vi "FM_pll.vi"() -> ()   [LabVIEW 2013]
uses:
  <vilib>/addons/Modulation/Analog/MT Passband PLL.vi
  <vilib>/sound2/lvsound2.llb/Sound File Info (path).vi
  <vilib>/sound2/lvsound2.llb/Sound File Read Open.vi
  <vilib>/sound2/lvsound2.llb/Sound File Read (DBL).vi
  <vilib>/Waveform/WDTOps.llb/WDT Get Waveform Subset DBL.vi
  <vilib>/express/express analysis/Spectral/Block/exnSpectralBlock spectral measurements RMS poly.vi
  <vilib>/express/express analysis/Spectral/Block/exnSpectralBlock spectral measurements RMS DDT.vi
  <vilib>/express/express analysis/Spectral/XNode/ExpressSpectralMeasurementsBlockNode.xnode
  <vilib>/addons/Modulation/niAMT.lvlib
  <vilib>/Analysis/NI_AALPro.lvlib
panel:
  in  "Modulated Signal Source":enum32{"Single Tone", "From File"}(tab)
  in  "ST Frequency":dbl=2000.0 caption="Frequency"
  in  "ST Amplitude":dbl=1.0 caption="Amplitude"
  in  "Resample Rate":dbl=1000000.0 format="%#_6f"
  in  "Duration":dbl=44100.0
  in  "WAV Path":path=path "E:/07/0409/mozart.wav" caption="Path"
  in  "Normalized Peak Amplitude":dbl=1.0 caption="Peak Amplitude"
  out "Estimated Freq.":dbl=100000.0 caption="Frequency"
  in  "WAV Sample Rate":dbl=44100.0 caption="dt"
  in  "LPF Cut-Off":dbl=20000.0 caption="Lower Cut-Off"
  in  "SNR (dB)":dbl(slide)=30.0 caption="Standard deviation" scale=-20.0..50.0
  out "Recovered Signal":dynamicdata(graph)
  out "Baseband":dynamicdata(graph)
  out "FM FFT":dynamicdata(graph)
  out "FM Wave":dynamicdata(graph)
  in  "Carrier Amp.":dbl=1.0 caption="Amplitude"
  in  "stop":bool
  in  "k_f":dbl(slide)=20000.0 scale=0.0..50000.0
  in  "Carrier Freq.":dbl=100000.0 caption="Frequency"
  # "Frequency Modulation"
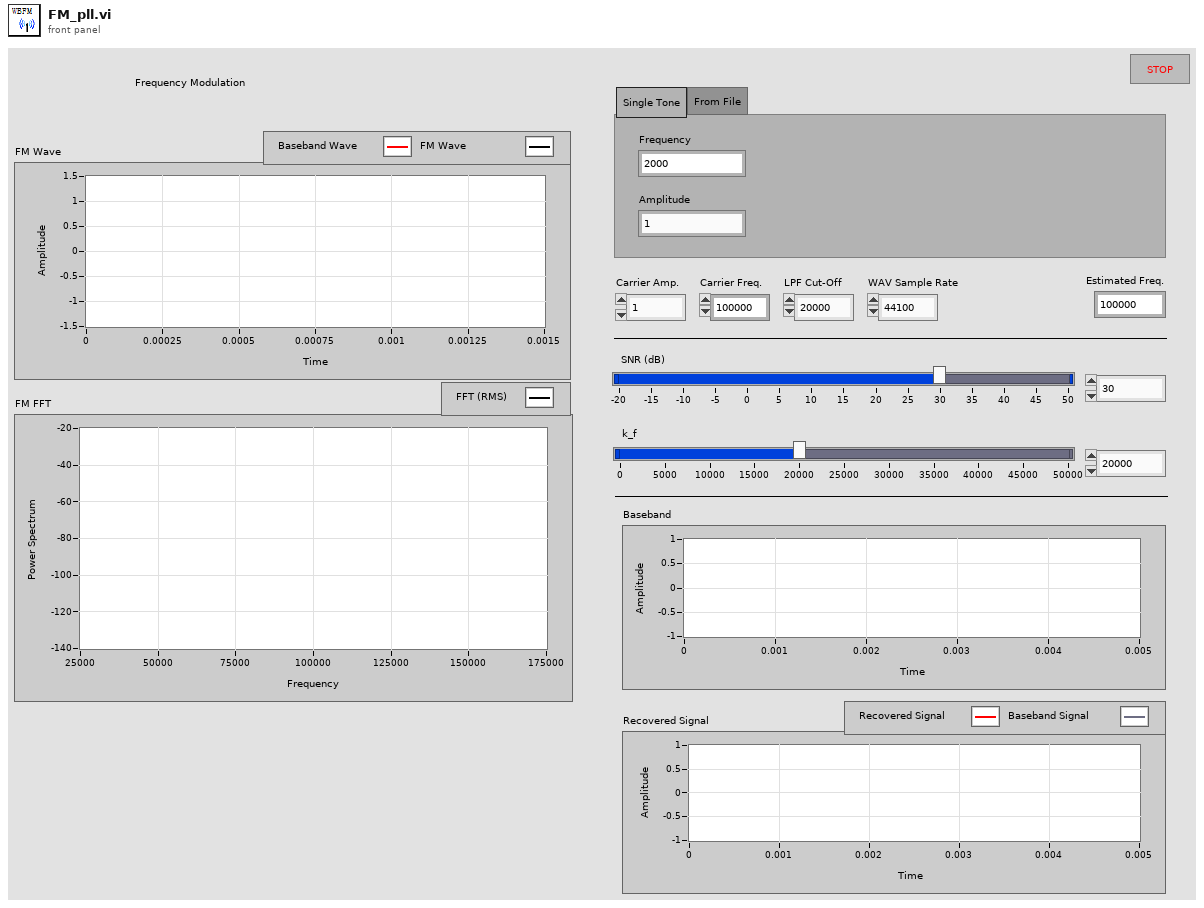
[diagram p1: front panel]
types:
  T1 = cluster{"averaging mode":u16, "weighting mode":u16, "number of averages":u32}
  T2 = cluster{"dB On (F)":bool, "unwrap phase (F)":bool, "convert to degree (F)":bool}
  T3 = typedef "Sound File Refnum.ctl" = refnum<file>
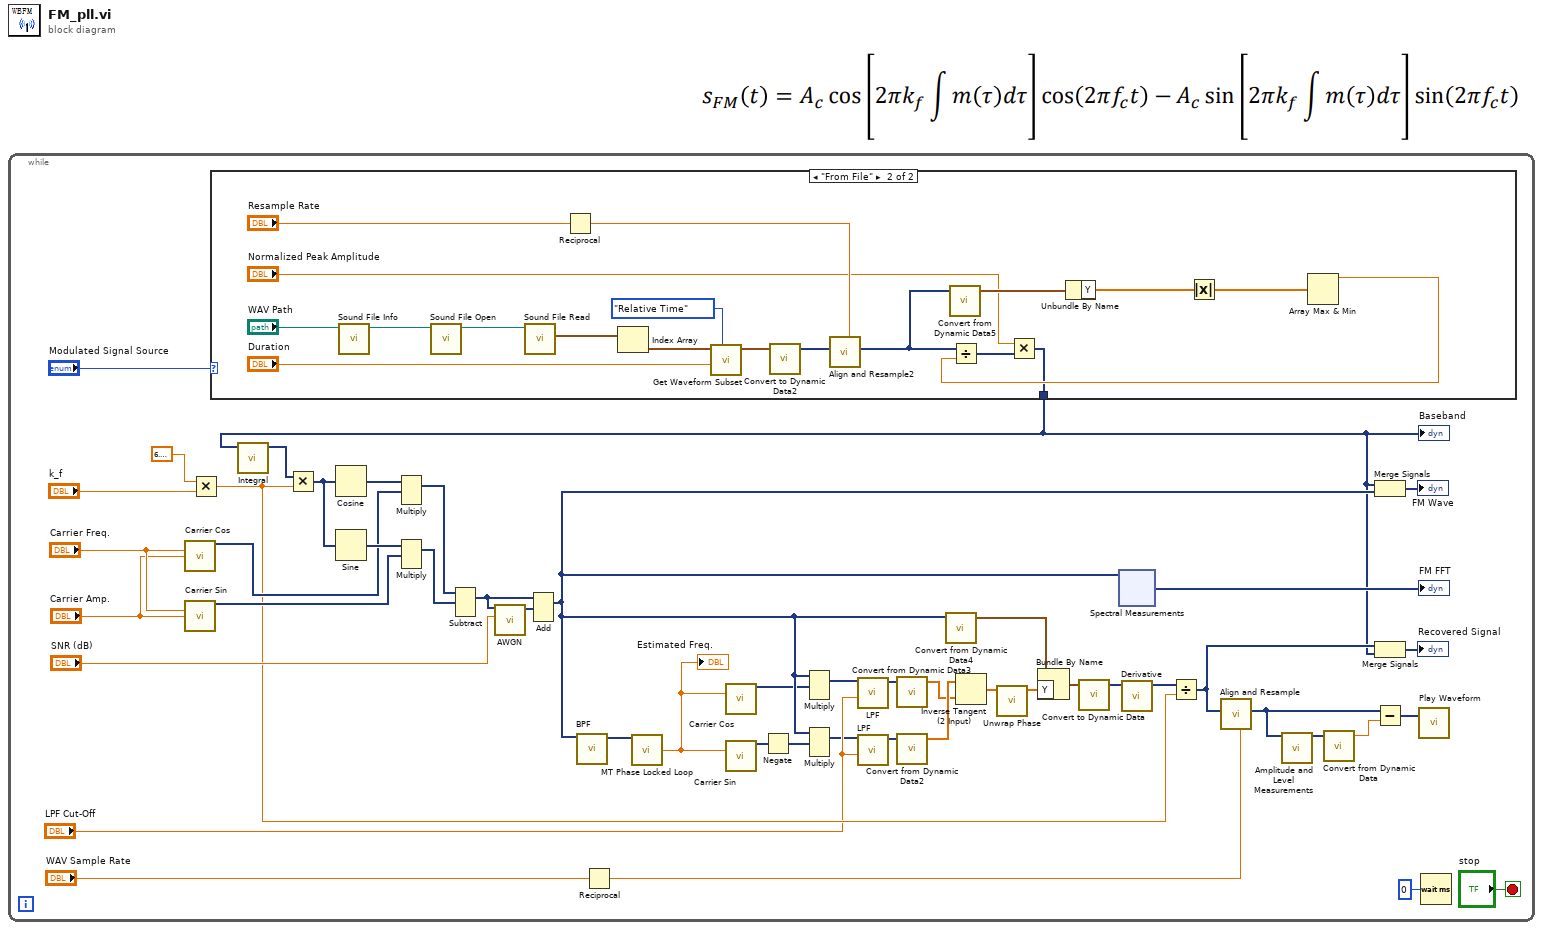
[diagram p0: block diagram]
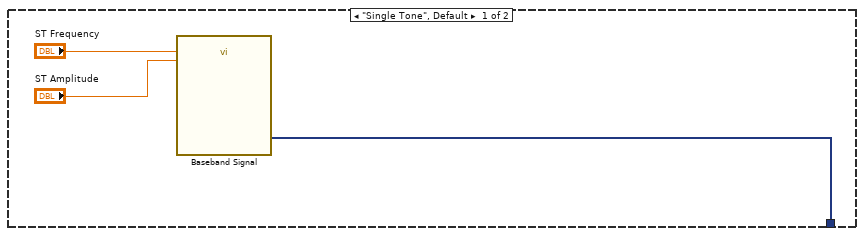
[diagram p2: hidden frame]
diagram:
  n1 = while {
    stop <- "stop" stop-if-true
    n2 = call "Carrier Cos"("Frequency"="Carrier Freq.", "Amplitude"="Carrier Amp.") -> ("Sine"=w28:dynamicdata)  [unwired: 12 in, 1 out]
    n3 = call "Carrier Sin"("Frequency"="Carrier Freq.", "Amplitude"="Carrier Amp.") -> ("Sine"=w27:dynamicdata)  [unwired: 12 in, 1 out]
    n4 = Multiply(x=6.283185307179586, y="k_f") -> (x*y=w23:dbl)
    n5 = case shown="\"From File\"" "Modulated Signal Source" {
      tunnel: [w50 w54] -> w1
      frame "Single Tone", Default {
        n6 = call "Baseband Signal"("Frequency"="ST Frequency", "Amplitude"="ST Amplitude") -> ("Sine"=w50:dynamicdata)  [unwired: 12 in, 1 out]
      }
      frame "From File" {
        n7 = call-poly <vilib>:"Sound File Info.vi"("path"="WAV Path") -> ("path out"=w69:path)  [unwired: 7 in, 3 out]
        n8 = call-poly <vilib>:"Sound File Open.vi"("path"=w69) -> ("sound file refnum"=w71:T3)  [unwired: 9 in, 1 out]
        n9 = call-poly <vilib>:"Sound File Read.vi"("sound file refnum"=w71) -> ("data"=w66:waveform(dbl)[])  [unwired: 6 in, 4 out]
        n10 = Reciprocal(x="Resample Rate") -> (1/x=w62:dbl)
        n11 = Index Array(array=w66) -> (element=w67:waveform(dbl))  [unwired: 1 in]
        n12 = call-poly <vilib>:"Get Waveform Subset.vi"("start/duration format"=enum16{"Relative Time"}."Relative Time", "duration"="Duration", "waveform in"=w67) -> ("waveform out"=w61:waveform(dbl))  [unwired: 3 in, 3 out]
        n13 = call "Convert to Dynamic Data2"("Waveform"=w61) -> ("Dynamic Data Type"=w56:dynamicdata)  [unwired: 3 in]
        n14 = call "Align and Resample2"("dt"=w62, "Signals"=w56) -> ("Resampled Signals"=w57:dynamicdata)  [unwired: 7 in, 2 out]
        n15 = call "Convert from Dynamic Data5"("Dynamic Data Type"=w57) -> ("Waveform"=w64:waveform(dbl))  [unwired: 3 in]
        n16 = Unbundle By Name(w64) -> ("Y"=w58:dbl[])
        n17 = Absolute Value(x=w58) -> (abs(x)=w60:dbl[])
        n18 = Array Max & Min(array=w60) -> (max value=w59:dbl)  [unwired: 3 out]
        n19 = Divide(x=w57, y=w59) -> (x/y=w55:dynamicdata)
        n20 = Multiply(x="Normalized Peak Amplitude", y=w55) -> (x*y=w54:dynamicdata)
      }
    }
    "Baseband" <- w1
    n21 = call "Integral"("Signals"=w1) -> ("Result"=w2:dynamicdata)  [unwired: 5 in, 1 out]
    n22 = Multiply(x=w2, y=w23) -> (x*y=w32:dynamicdata)
    n23 = Cosine(x=w32) -> (cos(x)=w34:dynamicdata)
    n24 = Sine(x=w32) -> (sin(x)=w33:dynamicdata)
    n25 = Multiply(1:w28, 2:w34) -> (0:w30:dynamicdata)  [unwired: 1 in, 1 out]
    n26 = Multiply(1:w27, 2:w33) -> (0:w29:dynamicdata)  [unwired: 1 in, 1 out]
    n27 = Subtract(1:w29, 2:w30) -> (0:w31:dynamicdata)  [unwired: 1 in, 1 out]
    n28 = call "AWGN.vi"("SNR (dB)"="SNR (dB)", "Dynamic Data"=w31) -> ("DC with Gaussian Noise"=w39:dynamicdata)  [unwired: 9 in]
    n29 = Add(1:w39, 2:w31) -> (0:w15:dynamicdata)  [unwired: 1 in, 1 out]
    n30 = call "BPF"("Signal"=w15) -> ("Filtered Signal"=w36:dynamicdata)  [unwired: 9 in, 1 out]
    n31 = Reciprocal(x="WAV Sample Rate") -> (1/x=w35:dbl)
    n32 = call-poly <vilib>:"MT Phase Locked Loop.vi"("passband waveform"=w36) -> ("estimated carrier frequency (Hz)"=w16:dbl)  [unwired: 10 in, 4 out]
    "Estimated Freq." <- w16
    n33 = call "Carrier Cos"("Frequency"=w16) -> ("Sine"=w13:dynamicdata)  [unwired: 13 in, 1 out]
    n34 = call "Carrier Sin"("Frequency"=w16) -> ("Sine"=w22:dynamicdata)  [unwired: 13 in, 1 out]
    n35 = Negate(x=w22) -> (-x=w14:dynamicdata)
    n36 = Multiply(1:w13, 2:w15) -> (0:w12:dynamicdata)  [unwired: 1 in, 1 out]
    n37 = Multiply(1:w14, 2:w15) -> (0:w11:dynamicdata)  [unwired: 1 in, 1 out]
    n38 = call "LPF"("Lower Cut-Off"="LPF Cut-Off", "Signal"=w12) -> ("Filtered Signal"=w19:dynamicdata)  [unwired: 8 in, 1 out]
    n39 = call "LPF"("Lower Cut-Off"="LPF Cut-Off", "Signal"=w11) -> ("Filtered Signal"=w20:dynamicdata)  [unwired: 8 in, 1 out]
    n40 = call "Convert from Dynamic Data3"("Dynamic Data Type"=w19) -> ("Array"=w17:dbl[])  [unwired: 3 in]
    n41 = call "Convert from Dynamic Data2"("Dynamic Data Type"=w20) -> ("Array"=w18:dbl[])  [unwired: 3 in]
    n42 = call "Convert from Dynamic Data4"("Dynamic Data Type"=w15) -> ("Waveform"=w9:waveform(dbl))  [unwired: 3 in]
    n43 = Inverse Tangent (2 Input)(1:w17, 2:w18) -> (0:w10:dbl[])
    n44 = call <vilib>:"Unwrap Phase.vi"("Phase"=w10) -> ("Unwrapped Phase"=w8:dbl[])  [unwired: 9 in, 1 out]
    n45 = Bundle By Name(cluster=w9, "Y"=w8) -> (w6:waveform(dbl))
    n46 = call "Convert to Dynamic Data"("Waveform"=w6) -> ("Dynamic Data Type"=w7:dynamicdata)  [unwired: 3 in]
    n47 = xnode ("Spectral Measurements")("Signals"=w15) -> ("FFT - (RMS)"=→"FM FFT":dynamicdata)  [unwired: 1 in, 2 out]
    n48 = call "Derivative"("Signals"=w7) -> ("Result"=w25:dynamicdata)  [unwired: 5 in, 1 out]
    n49 = Divide(x=w25, y=w23) -> (x/y=w24:dynamicdata)
    n50 = call "Align and Resample"("dt"=w35, "Signals"=w24) -> ("Resampled Signals"=w4:dynamicdata)  [unwired: 7 in, 2 out]
    n51 = call "Amplitude and Level Measurements"("Signals"=w4) -> ("Mean (DC)"=w45:dynamicdata)  [unwired: 13 in, 1 out]
    n52 = call "Convert from Dynamic Data"("Dynamic Data Type"=w45) -> ("Scalar"=w46:dbl)  [unwired: 3 in]
    n53 = Merge Signals(w1, w15) -> (→"FM Wave":dynamicdata)
    n54 = Merge Signals(w24, w1) -> (→"Recovered Signal":dynamicdata)
    n55 = Subtract(x=w4, y=w46) -> (x-y=w5:dynamicdata)
    n56 = call "Play Waveform"("Data"=w5) -> ()  [unwired: 18 in, 1 out]
    n57 = Wait (ms)(milliseconds to wait=u32 0) -> ()  [unwired: 1 out]
  }
